vi "Excel_Result.vi"(7 "Pass/Fail":bool, 8 "error in (no error)":errorcluster, 10 "Report path in":path) -> (0 "error out":errorcluster, 2 "Report path out":path)   [LabVIEW 2015]
doc: "在报表中显示本次测试是否通过"
uses:
  <vilib>/addons/_office/_exclsub.llb/font.ctl
  <vilib>/Utility/NIReport.llb/NI_report.lvclass
  <vilib>/addons/_office/NI_ReportGenerationToolkit.lvlib
panel:
  in  "start(-1,-1)":cluster{"row":i32, "column":i32}
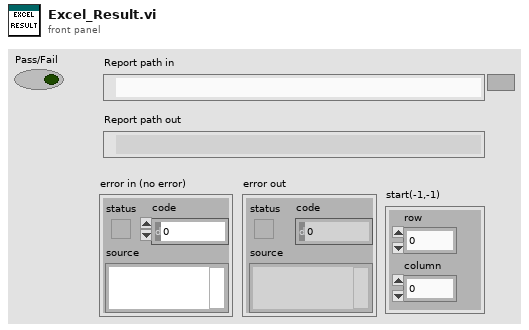
[diagram p1: front panel]
types:
  T1 = typedef "NI_ReportGenerationToolkit.lvlib/font.ctl" = cluster{"font name":string, "font size":dbl, "bold":u16, "italic":u16, "underline":u16, "strike through":u16, "font color":u32}
  T2 = enum16{"Standard Report", "HTML", "Word", "Excel"}
  T3 = enum16{"maximized", "minimized", "normal", "no change"}
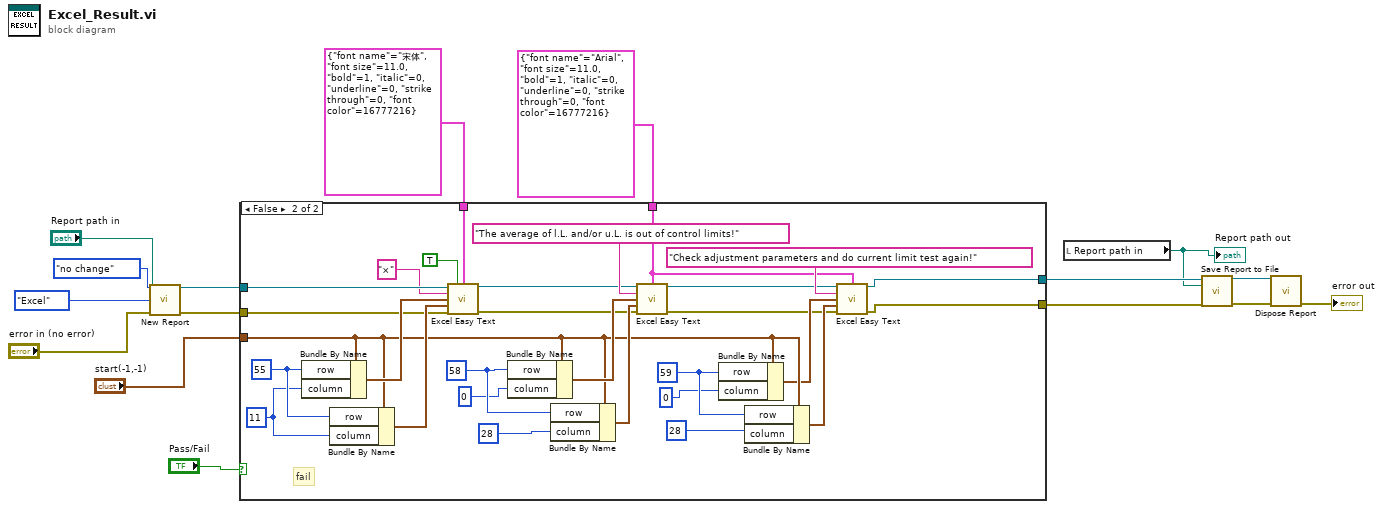
[diagram p0: block diagram]
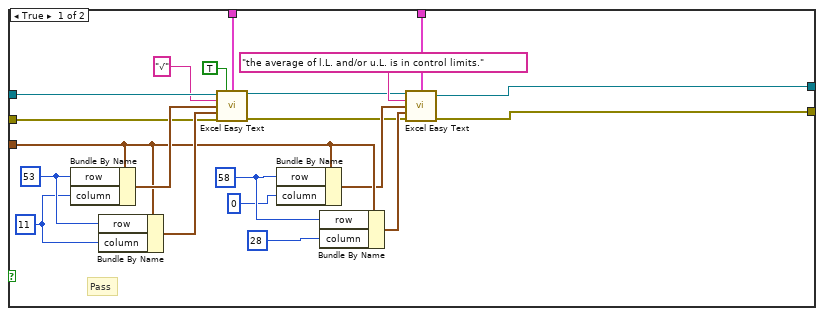
[diagram p2: hidden frame]
diagram:
  n1 = call <vilib>:"New Report.vi"("window state (normal)"=T3."no change", "report type"=T2."Excel", "template (empty)"="Report path in", "error in (no error)"="error in (no error)") -> ("report out"=w8:refnum<class "NI_report.lvclass">, "error out"=w7:errorcluster)  [unwired: 10 in]
  n2 = case shown="False" "Pass/Fail" {
    tunnel: "start(-1,-1)" -> [w31 w56]
    tunnel: T1 {"font name"="Arial", "font size"=11.0, "bold"=1, "italic"=0, "underline"=0, "strike through"=0, "font color"=16777216} ("font") -> [w32 w49]
    tunnel: w8 -> [w25 w48]
    tunnel: w7 -> [w24 w47]
    tunnel: [w21 w42] -> w6
    tunnel: [w20 w41] -> w5
    tunnel: T1 {"font name"="宋体", "font size"=11.0, "bold"=1, "italic"=0, "underline"=0, "strike through"=0, "font color"=16777216} ("font") -> [w19 w40]
    frame True {
      w28 = 58 ("row")
      w35 = 11 ("row")
      w36 = 53 ("row")
      # "Pass"
      n3 = Bundle By Name(cluster=w31, "row"=w36, "column"=w35) -> (w37:cluster{"row":i32, "column":i32})
      n4 = Bundle By Name(cluster=w31, "row"=w36, "column"=w35) -> (w34:cluster{"row":i32, "column":i32})
      n5 = call <vilib>:"Excel Easy Text.vi"("report in"=w25, "border? (F)"=TRUE, "font"=w19, "text"="√", "start (-1, -1)"=w37, "end (-1, -1)"=w34, "error in (no error)"=w24) -> ("report out"=w23:refnum<class "NI_report.lvclass">, "error out"=w22:errorcluster)  [unwired: 4 in, 3 out]
      n6 = Bundle By Name(cluster=w31, "row"=w28, "column"=0) -> (w30:cluster{"row":i32, "column":i32})
      n7 = Bundle By Name(cluster=w31, "row"=w28, "column"=28) -> (w29:cluster{"row":i32, "column":i32})
      n8 = call <vilib>:"Excel Easy Text.vi"("report in"=w23, "font"=w32, "text"="the average of l.L. and/or u.L. is in control limits.", "start (-1, -1)"=w30, "end (-1, -1)"=w29, "error in (no error)"=w22) -> ("report out"=w21:refnum<class "NI_report.lvclass">, "error out"=w20:errorcluster)  [unwired: 5 in, 3 out]
    }
    frame False {
      w53 = 59 ("row")
      w59 = 58 ("row")
      w64 = 11 ("row")
      w65 = 55 ("row")
      # "fail"
      n9 = Bundle By Name(cluster=w56, "row"=w65, "column"=w64) -> (w66:cluster{"row":i32, "column":i32})
      n10 = Bundle By Name(cluster=w56, "row"=w65, "column"=w64) -> (w63:cluster{"row":i32, "column":i32})
      n11 = call <vilib>:"Excel Easy Text.vi"("report in"=w48, "border? (F)"=TRUE, "font"=w40, "text"="×", "start (-1, -1)"=w66, "end (-1, -1)"=w63, "error in (no error)"=w47) -> ("report out"=w46:refnum<class "NI_report.lvclass">, "error out"=w45:errorcluster)  [unwired: 4 in, 3 out]
      n12 = Bundle By Name(cluster=w56, "row"=w59, "column"=0) -> (w61:cluster{"row":i32, "column":i32})
      n13 = Bundle By Name(cluster=w56, "row"=w59, "column"=28) -> (w60:cluster{"row":i32, "column":i32})
      n14 = call <vilib>:"Excel Easy Text.vi"("report in"=w46, "font"=w49, "text"="The average of l.L. and/or u.L. is out of control limits!", "start (-1, -1)"=w61, "end (-1, -1)"=w60, "error in (no error)"=w45) -> ("report out"=w44:refnum<class "NI_report.lvclass">, "error out"=w43:errorcluster)  [unwired: 5 in, 3 out]
      n15 = Bundle By Name(cluster=w56, "row"=w53, "column"=0) -> (w55:cluster{"row":i32, "column":i32})
      n16 = Bundle By Name(cluster=w56, "row"=w53, "column"=28) -> (w54:cluster{"row":i32, "column":i32})
      n17 = call <vilib>:"Excel Easy Text.vi"("report in"=w44, "font"=w49, "text"="Check adjustment parameters and do current limit test again!", "start (-1, -1)"=w55, "end (-1, -1)"=w54, "error in (no error)"=w43) -> ("report out"=w42:refnum<class "NI_report.lvclass">, "error out"=w41:errorcluster)  [unwired: 5 in, 3 out]
    }
  }
  n18 = local read "Report path in"() -> (w2:path)
  "Report path out" <- w2
  n19 = call-dynamic "Save Report to File.vi"("report in"=w6, "report file path"=w2, "error in (no error)"=w5) -> ("report out"=w4:refnum<class "NI_report.lvclass">, "error out"=w3:errorcluster)  [unwired: 11 in]
  n20 = call-dynamic "Dispose Report.vi"("report in"=w4, "error in (no error)"=w3) -> ("error out"=→"error out":errorcluster)  [unwired: 13 in]
